vi "CheckROIBoundary.vi"(8 "error in (no error)":errorcluster, 11 "Camera in":refnum<class "Camera.lvclass">) -> (0 "error out":errorcluster, 2 "Valid?":bool, 3 "Camera out":refnum<class "Camera.lvclass">)   [LabVIEW 2020, in "Camera.lvlib" / "Camera.lvclass"]
uses:
  Camera.lvclass
  Camera.lvclass/Camera.ctl
panel:
  in  "Full CCD Height":u16
  in  "Full CCD Width":u16
  in  "Height":u16
  in  "Y":u16
  in  "Width":u16
  in  "X":u16
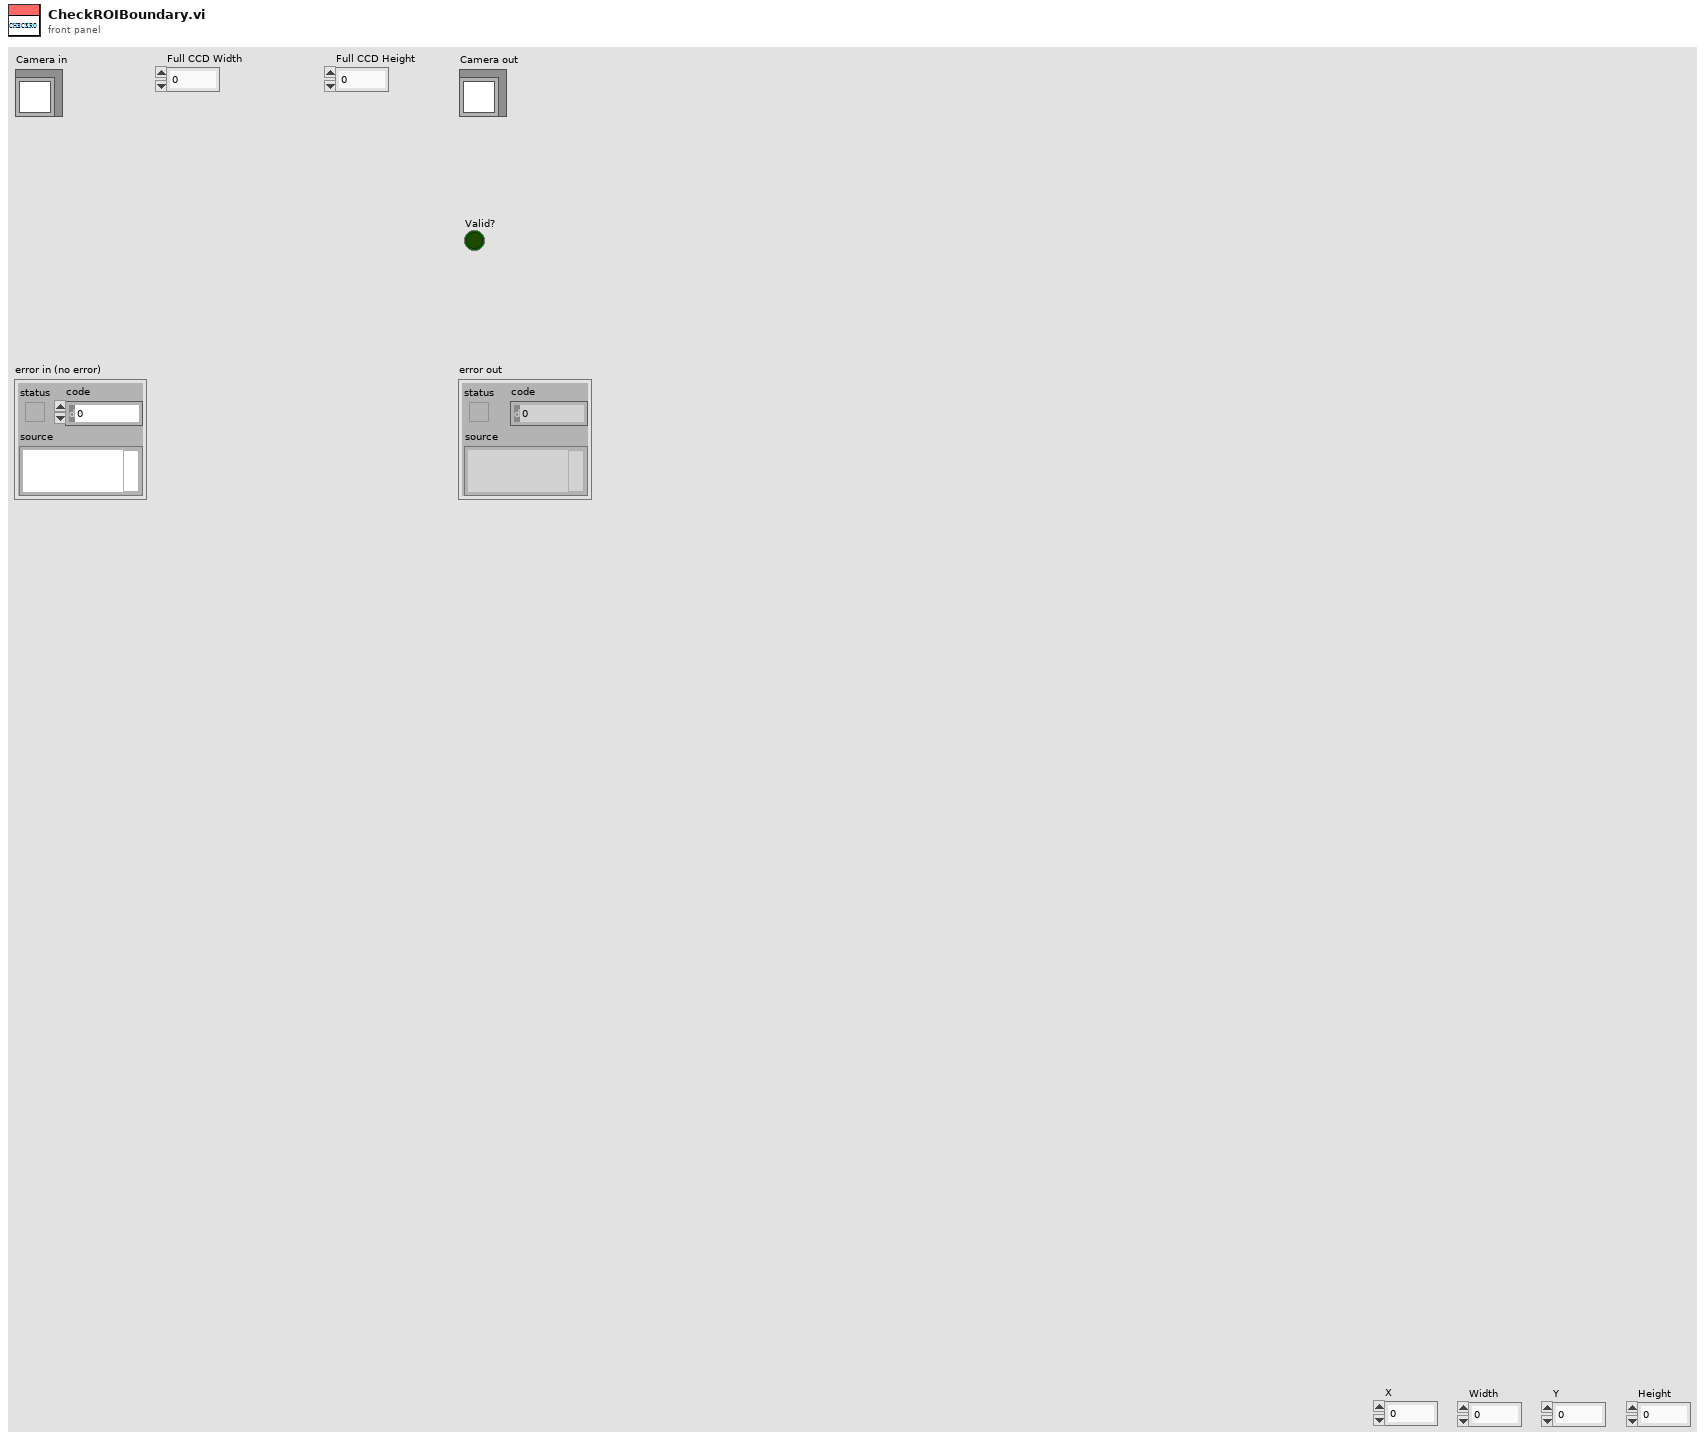
[diagram p1: front panel]
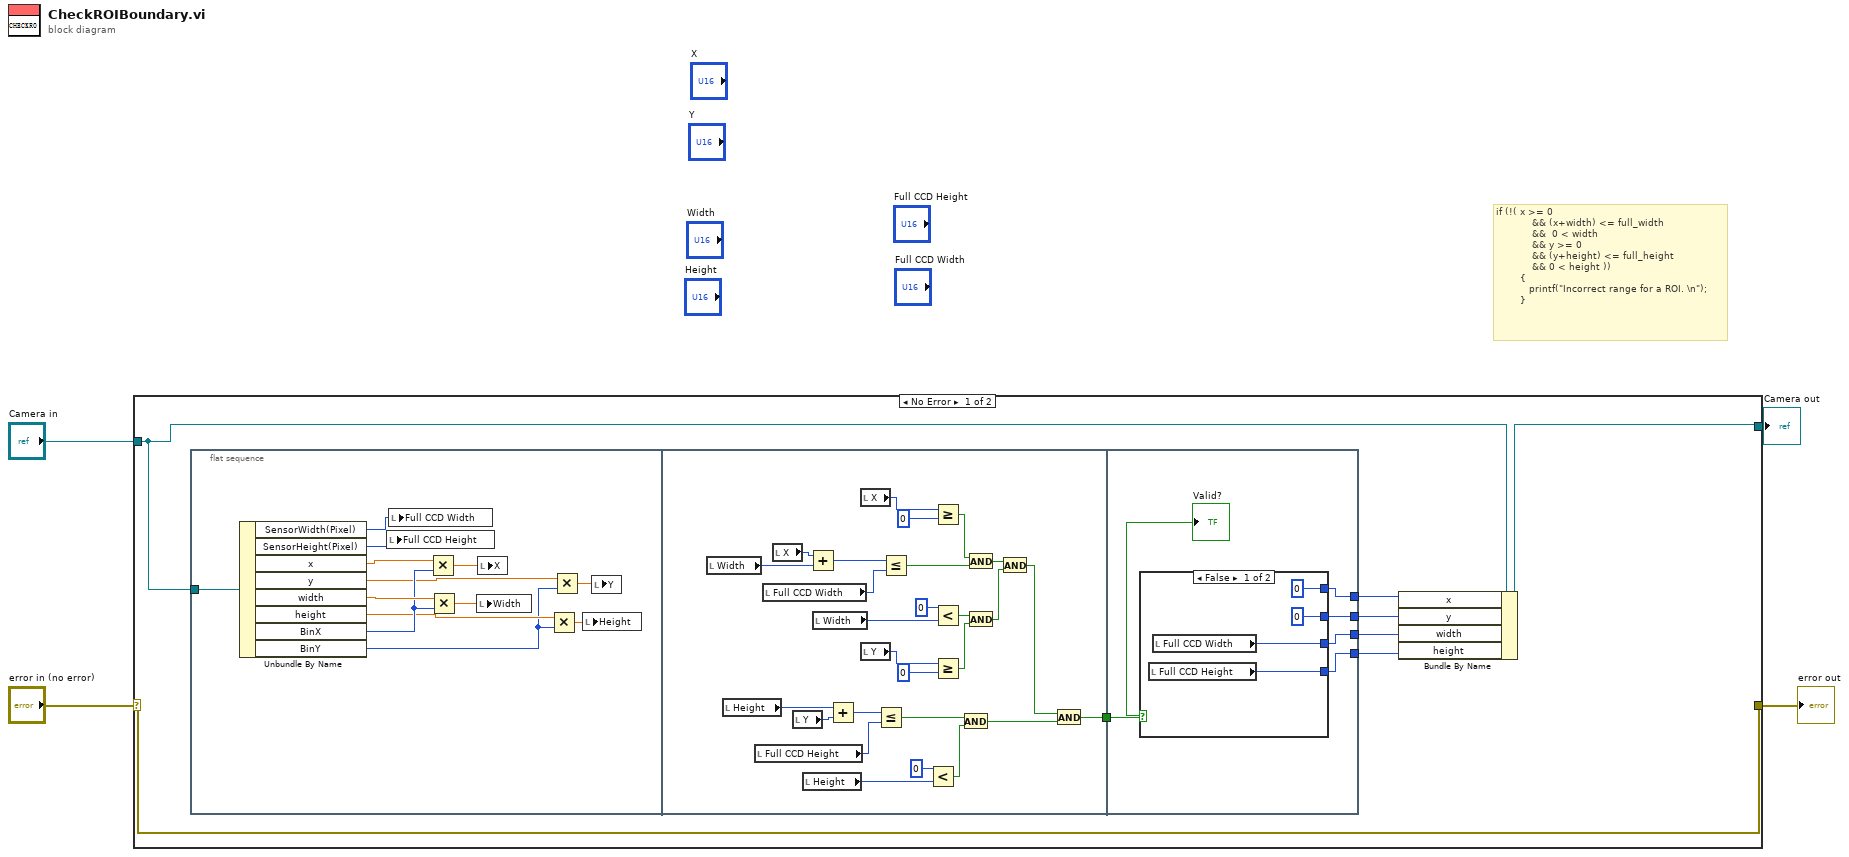
[diagram p0: block diagram]
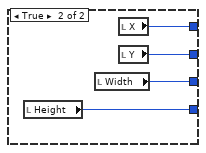
[diagram p2: hidden frame]
diagram:
  # "if (!( x >= 0\n            && (x+width) <= full_width\n            &&  0 < width \n            && y >= 0\n            && (y+height) <= full_height\n            && 0 < height ))\n        {\n           printf(\"Incorrect range for a ROI. \\n\");\n        }"
  n1 = case shown="No Error" "error in (no error)" {
    selector: "error in (no error)" -> [w12 w67]
    tunnel: [w12 w67] -> w3
    tunnel: [w9 w66] -> w1
    tunnel: "Camera in" -> [w11 w66]
    frame No Error {
      n2 = flat-sequence {
        tunnel: w11 -> [w25]
        tunnel: [w26] -> w10
        tunnel: w10 -> [w57]
        tunnel: [w56] -> w8
        tunnel: [w55] -> w7
        tunnel: [w54] -> w6
        tunnel: [w53] -> w5
        frame #0 {
          n3 = Unbundle By Name(w25) -> ("SensorWidth(Pixel)"=w23:i32, "SensorHeight(Pixel)"=w24:i32, "x"=w22:dbl, "y"=w17:dbl, "width"=w21:dbl, "height"=w16:dbl, "BinX"=w20:i32, "BinY"=w15:i32)
          n4 = local write "Full CCD Height"(w24) -> ()
          n5 = local write "Full CCD Width"(w23) -> ()
          n6 = Multiply(x=w22, y=w20) -> (x*y=w19:dbl)
          n7 = Multiply(x=w21, y=w20) -> (x*y=w18:dbl)
          n8 = local write "Width"(w18) -> ()
          n9 = local write "X"(w19) -> ()
          n10 = Multiply(x=w16, y=w15) -> (x*y=w13:dbl)
          n11 = Multiply(x=w17, y=w15) -> (x*y=w14:dbl)
          n12 = local write "Height"(w13) -> ()
          n13 = local write "Y"(w14) -> ()
        }
        frame #1 {
          n14 = local read "Width"() -> (w40:u16)
          n15 = local read "Height"() -> (w38:u16)
          n16 = local read "Full CCD Height"() -> (w34:u16)
          n17 = local read "Full CCD Width"() -> (w36:u16)
          n18 = local read "X"() -> (w41:u16)
          n19 = local read "Y"() -> (w37:u16)
          n20 = local read "Height"() -> (w31:u16)
          n21 = Add(x=w41, y=w40) -> (x+y=w35:u16)
          n22 = local read "Width"() -> (w32:u16)
          n23 = Add(x=w38, y=w37) -> (x+y=w33:u16)
          n24 = local read "X"() -> (w42:u16)
          n25 = local read "Y"() -> (w39:u16)
          n26 = Less Or Equal?(x=w33, y=w34) -> (x <= y?=w48:bool)
          n27 = Less Or Equal?(x=w35, y=w36) -> (x <= y?=w51:bool)
          n28 = Less?(x=u16 0 ("y"), y=w31) -> (x < y?=w47:bool)
          n29 = Greater Or Equal?(x=w42, y=u16 0) -> (x >= y?=w52:bool)
          n30 = Less?(x=u16 0 ("y"), y=w32) -> (x < y?=w50:bool)
          n31 = Greater Or Equal?(x=w39, y=u16 0) -> (x >= y?=w49:bool)
          n32 = And(x=w48, y=w47) -> (x .and. y?=w43:bool)
          n33 = And(x=w52, y=w51) -> (x .and. y?=w46:bool)
          n34 = And(x=w50, y=w49) -> (x .and. y?=w45:bool)
          n35 = And(x=w46, y=w45) -> (x .and. y?=w44:bool)
          n36 = And(x=w44, y=w43) -> (x .and. y?=w26:bool)
        }
        frame #2 {
          n37 = case shown="False" w57 {
            tunnel: [w58 w65] -> w54
            tunnel: [u16 0 ("X") w64] -> w56
            tunnel: [u16 0 ("Y") w63] -> w55
            tunnel: [w59 w62] -> w53
            frame False {
              n38 = local read "Full CCD Height"() -> (w59:u16)
              n39 = local read "Full CCD Width"() -> (w58:u16)
            }
            frame True {
              n40 = local read "Height"() -> (w62:u16)
              n41 = local read "Width"() -> (w65:u16)
              n42 = local read "X"() -> (w64:u16)
              n43 = local read "Y"() -> (w63:u16)
            }
          }
          "Valid?" <- w57
        }
      }
      n44 = Bundle By Name(cluster=w11, "x"=w8, "y"=w7, "width"=w6, "height"=w5) -> (w9:refnum<class "Camera.lvclass">)
    }
    frame Error {
    }
  }
  "error out" <- w3
  "Camera out" <- w1
